vi "Update Value Control.vi"(0 "Session In":T2, 5 "Active Item:Tag":string, 7 "Tab Control Ref In":T1, 11 "error in (no error)":errorcluster) -> (4 "Session Out":T2, 15 "error out":errorcluster)   [LabVIEW 2014, in "Camera Quick Settings Panel.lvlib" / "Camera Quick Settings Panel.lvclass"]
doc: "The Update Value Control subVI determines the type of the attribute selected, displays the corresponding tab in the tab control, sets the current value of the control, sets the minimum and maximum of the control (for numerics), and disables the control if the attribute is not writables."
uses:
  Camera Quick Settings Panel.lvclass
  <vilib>/userdefined/High Color/IMAQdx.ctl
  <vilib>/vision/driver/IMAQdx.llb/IMAQdx Attribute Type.ctl
  <vilib>/vision/driver/NI_Vision_Acquisition_Software.lvlib
  <resource>/objmgr/imaqdx.rc
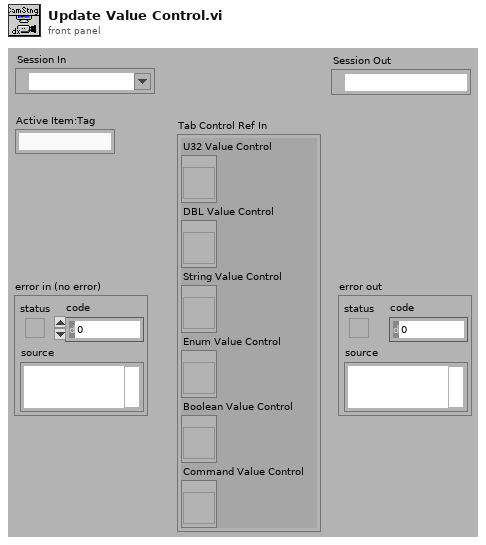
[diagram p1: front panel]
types:
  T1 = cluster{"U32 Value Control":refnum<vi>, "DBL Value Control":refnum<vi>, "String Value Control":refnum<vi>, "Enum Value Control":refnum<vi>, "Boolean Value Control":refnum<vi>, "Command Value Control":refnum<vi>}
  T2 = typedef "IMAQdx.ctl" = refnum<k21>
  T3 = typedef "NI_Vision_Acquisition_Software.lvlib/IMAQdx Attribute Type.ctl" = enum32{"U32", "I64", "DBL", "String", "Enum", "Bool", "Command"}
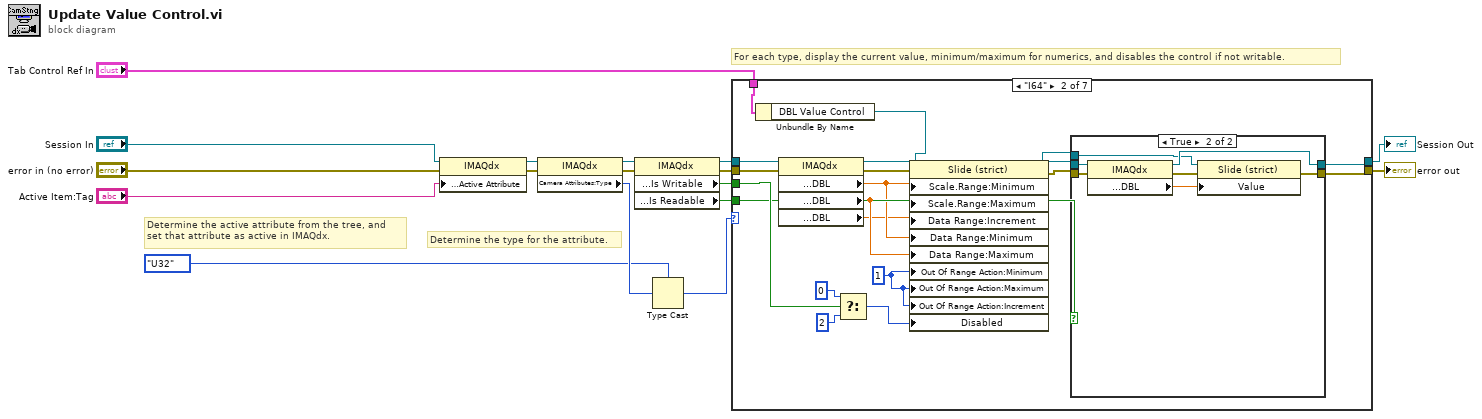
[diagram p0: block diagram]
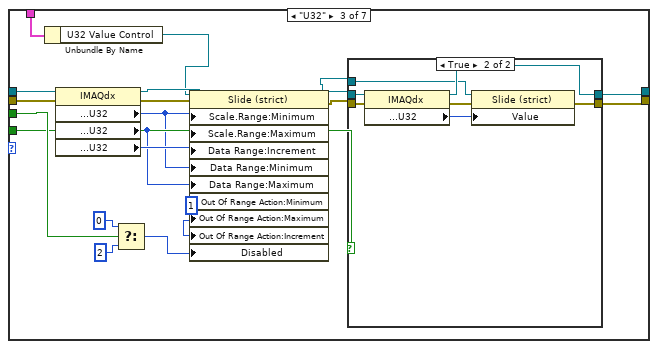
[diagram p4: hidden frame]
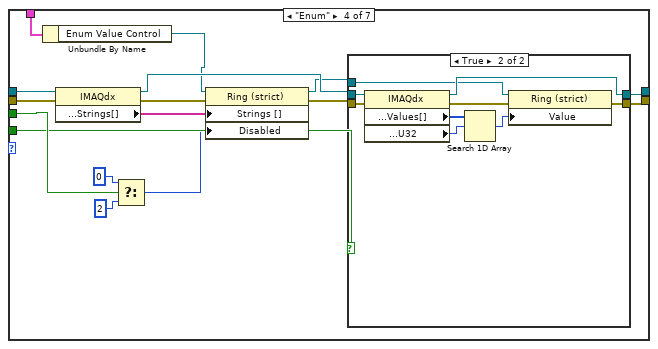
[diagram p6: hidden frame]
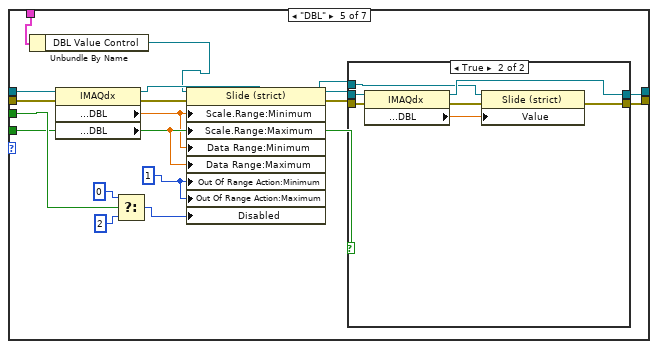
[diagram p8: hidden frame]
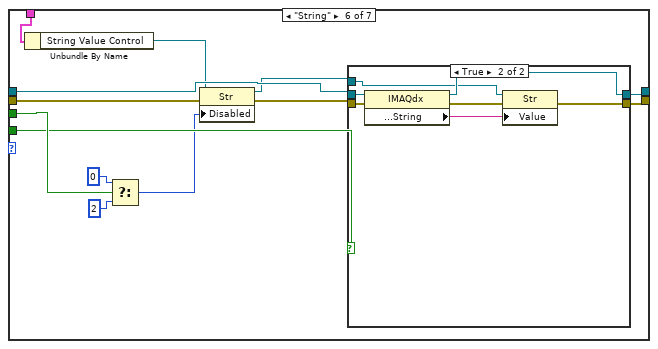
[diagram p10: hidden frame]
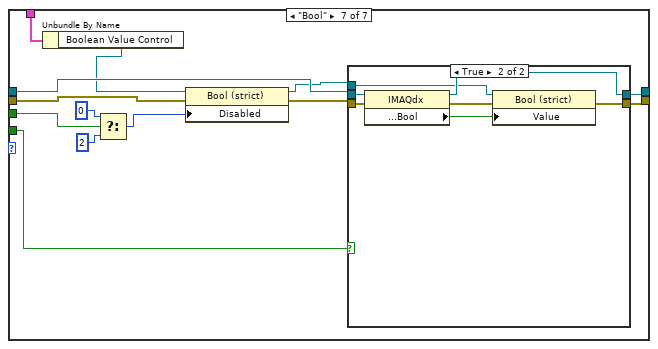
[diagram p12: hidden frame]
diagram:
  # "For each type, display the current value, minimum/maximum for numerics, and disables the control if not writable."
  # "Determine the type for the attribute."
  # "Determine the active attribute from the tree, and \nset that attribute as active in IMAQdx."
  n1 = property class="IMAQdx"(reference="Session In", error in="error in (no error)", "Camera Attributes:Active Attribute"="Active Item:Tag") -> (reference out=w17:T2, error out=w16:errorcluster)
  n2 = property class="IMAQdx"(reference=w17, error in=w16) -> (reference out=w14:T2, error out=w15:errorcluster, "Camera Attributes:Type"=w6:u32)
  n3 = property class="IMAQdx"(reference=w14, error in=w15) -> (reference out=w2:T2, error out=w1:errorcluster, "Camera Attributes:Is Writable"=w4:bool, "Camera Attributes:Is Readable"=w3:bool)
  n4 = Type Cast(type=IMAQdx_Attribute_Type."U32" ("Attribute Type"), x=w6) -> (*(type *) &x=w13:T3)
  n5 = case shown="\"I64\"" w13 {
    tunnel: w4 -> [_ w36 w64 w89 w118 w141 w162]
    tunnel: w3 -> [_ w35 w63 w88 w117 w140 w164]
    tunnel: w2 -> [w18 w38 w66 w91 w120 w139 w161]
    tunnel: w1 -> [w19 w37 w65 w90 w119 w142 w163]
    tunnel: [w19 w32 w60 w85 w114 w137 w159] -> w9
    tunnel: [w18 w31 w59 w84 w113 w136 w158] -> w10
    tunnel: "Tab Control Ref In" -> [_ w30 w57 w82 w112 w135 w157]
    frame "Command" {
    }
    frame "I64" {
      w21 = u8 1 ("Out Of Range Action:Maximum")
      n6 = Unbundle By Name(w30) -> ("DBL Value Control"=w29:refnum<vi>)
      n7 = property class="IMAQdx"(reference=w38, error in=w37) -> (reference out=w34:T2, error out=w25:errorcluster, "Camera Attributes:Minimum:DBL"=w23:dbl, "Camera Attributes:Maximum:DBL"=w22:dbl, "Camera Attributes:Increment:DBL"=w20:dbl)
      n8 = Select(t=0, s=w36, f=2) -> (s? t:f=w24:i32)
      n9 = property class="Slide (strict)"(reference=w29, error in=w25, "Scale.Range:Minimum"=w23, "Scale.Range:Maximum"=w22, "Data Range:Increment"=w20, "Data Range:Minimum"=w23, "Data Range:Maximum"=w22, "Out Of Range Action:Minimum"=w21, "Out Of Range Action:Maximum"=w21, "Out Of Range Action:Increment"=w21, "Disabled"=w24) -> (reference out=w28:refnum<vi>, error out=w33:errorcluster)
      n10 = case shown="True" w35 {
        tunnel: w34 -> [w40 w47]
        tunnel: w33 -> [w39 w46]
        tunnel: [w40 w44] -> w31
        tunnel: [w39 w45] -> w32
        tunnel: w28 -> [_ w42]
        frame False {
        }
        frame True {
          n11 = property class="IMAQdx"(reference=w47, error in=w46) -> (reference out=w44:T2, error out=w43:errorcluster, "Camera Attributes:Value:DBL"=w41:dbl)
          n12 = property class="Slide (strict)"(reference=w42, error in=w43, "Value"=w41) -> (error out=w45:errorcluster)  [unwired: 1 out]
        }
      }
    }
    frame "U32" {
      w51 = u8 1 ("Out Of Range Action:Maximum")
      n13 = Unbundle By Name(w57) -> ("U32 Value Control"=w56:refnum<vi>)
      n14 = property class="IMAQdx"(reference=w66, error in=w65) -> (reference out=w62:T2, error out=w53:errorcluster, "Camera Attributes:Minimum:U32"=w49:u32, "Camera Attributes:Maximum:U32"=w48:u32, "Camera Attributes:Increment:U32"=w50:u32)
      n15 = Select(t=0, s=w64, f=2) -> (s? t:f=w52:i32)
      n16 = property class="Slide (strict)"(reference=w56, error in=w53, "Scale.Range:Minimum"=w49, "Scale.Range:Maximum"=w48, "Data Range:Increment"=w50, "Data Range:Minimum"=w49, "Data Range:Maximum"=w48, "Out Of Range Action:Minimum"=w51, "Out Of Range Action:Maximum"=w51, "Out Of Range Action:Increment"=w51, "Disabled"=w52) -> (reference out=w58:refnum<vi>, error out=w61:errorcluster)
      n17 = case shown="True" w63 {
        tunnel: w62 -> [w68 w75]
        tunnel: w61 -> [w67 w74]
        tunnel: [w68 w73] -> w59
        tunnel: [w67 w69] -> w60
        tunnel: w58 -> [_ w70]
        frame False {
        }
        frame True {
          n18 = property class="IMAQdx"(reference=w75, error in=w74) -> (reference out=w73:T2, error out=w72:errorcluster, "Camera Attributes:Value:U32"=w71:u32)
          n19 = property class="Slide (strict)"(reference=w70, error in=w72, "Value"=w71) -> (error out=w69:errorcluster)  [unwired: 1 out]
        }
      }
    }
    frame "Enum" {
      n20 = Unbundle By Name(w82) -> ("Enum Value Control"=w81:refnum<vi>)
      n21 = property class="IMAQdx"(reference=w91, error in=w90) -> (reference out=w87:T2, error out=w78:errorcluster, "Camera Attributes:Enum:Strings[]"=w76:string[])
      n22 = Select(t=0, s=w89, f=2) -> (s? t:f=w77:i32)
      n23 = property class="Ring (strict)"(reference=w81, error in=w78, "Strings []"=w76, "Disabled"=w77) -> (reference out=w83:refnum<vi>, error out=w86:errorcluster)
      n24 = case shown="True" w88 {
        tunnel: w87 -> [w93 w102]
        tunnel: w86 -> [w92 w101]
        tunnel: [w93 w96] -> w84
        tunnel: [w92 w98] -> w85
        tunnel: w83 -> [_ w95]
        frame False {
        }
        frame True {
          n25 = property class="IMAQdx"(reference=w102, error in=w101) -> (reference out=w96:T2, error out=w94:errorcluster, "Camera Attributes:Enum:Values[]"=w100:u32[], "Camera Attributes:Value:U32"=w99:u32)
          n26 = Search 1D Array(1D array=w100, element=w99) -> (index of element=w97:i32)  [unwired: 1 out]
          n27 = property class="Ring (strict)"(reference=w95, error in=w94, "Value"=w97) -> (error out=w98:errorcluster)  [unwired: 1 out]
        }
      }
    }
    frame "DBL" {
      w103 = u8 1 ("Out Of Range Action:Minimum")
      n28 = Unbundle By Name(w112) -> ("DBL Value Control"=w111:refnum<vi>)
      n29 = property class="IMAQdx"(reference=w120, error in=w119) -> (reference out=w116:T2, error out=w107:errorcluster, "Camera Attributes:Minimum:DBL"=w105:dbl, "Camera Attributes:Maximum:DBL"=w104:dbl)
      n30 = Select(t=0, s=w118, f=2) -> (s? t:f=w106:i32)
      n31 = property class="Slide (strict)"(reference=w111, error in=w107, "Scale.Range:Minimum"=w105, "Scale.Range:Maximum"=w104, "Data Range:Minimum"=w105, "Data Range:Maximum"=w104, "Out Of Range Action:Minimum"=w103, "Out Of Range Action:Maximum"=w103, "Disabled"=w106) -> (reference out=w110:refnum<vi>, error out=w115:errorcluster)
      n32 = case shown="True" w117 {
        tunnel: w116 -> [w122 w129]
        tunnel: w115 -> [w121 w128]
        tunnel: [w122 w127] -> w113
        tunnel: [w121 w125] -> w114
        tunnel: w110 -> [_ w124]
        frame False {
        }
        frame True {
          n33 = property class="IMAQdx"(reference=w129, error in=w128) -> (reference out=w127:T2, error out=w126:errorcluster, "Camera Attributes:Value:DBL"=w123:dbl)
          n34 = property class="Slide (strict)"(reference=w124, error in=w126, "Value"=w123) -> (error out=w125:errorcluster)  [unwired: 1 out]
        }
      }
    }
    frame "String" {
      n35 = Unbundle By Name(w135) -> ("String Value Control"=w134:refnum<vi>)
      n36 = Select(t=0, s=w141, f=2) -> (s? t:f=w130:i32)
      n37 = property class="Str"(reference=w134, error in=w142, "Disabled"=w130) -> (reference out=w133:refnum<vi>, error out=w138:errorcluster)
      n38 = case shown="True" w140 {
        tunnel: w139 -> [w144 w151]
        tunnel: w138 -> [w143 w150]
        tunnel: [w144 w149] -> w136
        tunnel: [w143 w147] -> w137
        tunnel: w133 -> [_ w145]
        frame False {
        }
        frame True {
          n39 = property class="IMAQdx"(reference=w151, error in=w150) -> (reference out=w149:T2, error out=w148:errorcluster, "Camera Attributes:Value:String"=w146:string)
          n40 = property class="Str"(reference=w145, error in=w148, "Value"=w146) -> (error out=w147:errorcluster)  [unwired: 1 out]
        }
      }
    }
    frame "Bool" {
      n41 = Unbundle By Name(w157) -> ("Boolean Value Control"=w156:refnum<vi>)
      n42 = Select(t=0, s=w162, f=2) -> (s? t:f=w152:i32)
      n43 = property class="Bool (strict)"(reference=w156, error in=w163, "Disabled"=w152) -> (reference out=w155:refnum<vi>, error out=w160:errorcluster)
      n44 = case shown="True" w164 {
        tunnel: w161 -> [w166 w173]
        tunnel: w160 -> [w165 w172]
        tunnel: [w166 w171] -> w158
        tunnel: [w165 w169] -> w159
        tunnel: w155 -> [_ w167]
        frame False {
        }
        frame True {
          n45 = property class="IMAQdx"(reference=w173, error in=w172) -> (reference out=w171:T2, error out=w170:errorcluster, "Camera Attributes:Value:Bool"=w168:bool)
          n46 = property class="Bool (strict)"(reference=w167, error in=w170, "Value"=w168) -> (error out=w169:errorcluster)  [unwired: 1 out]
        }
      }
    }
  }
  "Session Out" <- w10
  "error out" <- w9
